vi "Regler Druck Kalter Block.vi"(7 "Index":i32, 8 "Fehler":errorcluster caption="Fehler (Eingang)") -> (0 "Fehler (Ausgang)":errorcluster)   [LabVIEW 2020, in "Regler.lvlib" / "Druckregler.lvlib"]
uses:
  Druckregler.lvlib
  Aktionen Param. Druckregler.ctl
  Aktionen Interne Werte.ctl
  Verwaltung/FGV IN Aktionen.ctl
  Konfig-Dateien/FGV Betriebsdaten Aktionen.ctl
  Verwaltung/FGV OUT Aktionen.ctl
  Allgemein/Aktionen FGV Dichtheitstest.ctl
  Allgemein/FGV Zustaende Aktionen.ctl
  Funktionstasten/Zustaende.ctl
  Allgemein/FGV Analysator aktiv.ctl
  Seiten/CalGas Aufschaltung/Auswahl Analysator.ctl
  Seiten/CalGas Aufschaltung/Auswahl Aufschaltpunkt.ctl
  Verwaltung/Verwaltung - cRIO.lvlib
  Visualisierungs Elemente/Zahlen-Eingabefeld.ctl
  Allgemein/Allgemein.lvlib
  Konfig-Dateien/Konfig-Dateien.lvlib
  Funktionstasten/Funktionstasten.lvlib
  Seiten/CalGas Aufschaltung/CalGas Aufschaltung.lvlib
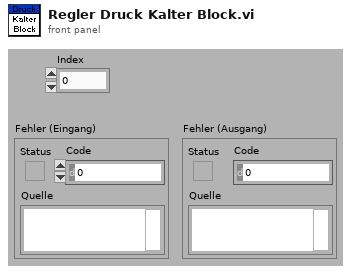
[diagram p1: front panel]
types:
  T1 = typedef "Regler.lvlib/Druckregler.lvlib/Aktionen Param. Druckregler.ctl" = enum16{"lesen", "schreiben", "Regler FT-IR", "Regler Ausgang", "Regler Durchfluss", "Regler PMA", "Regler NDIR", "Regler Filterblock", "Regler Gaskühler", "Regler Kalter Block"}
  T2 = typedef "Allgemein.lvlib/FGV Analysator aktiv.ctl" = enum16{"lesen", "Analysator", "CG Aufschaltung", "KAL Zustand", "AutaKal GT?"}
  T3 = typedef "Funktionstasten.lvlib/Zustaende.ctl" = enum16{"Standby", "Pause", "Eco", "Messen", "Kalibrieren", "Spülen Filter", "Spülen Leitung", "Umgebungsluft", "0-Gas", "Cal-Gas", "CG zu PNS", "-------------", "Init 1", "Init 2", "Init 3", "Init 4", "Messen vorbereiten", "Messen durchführen", "Exit"}
  T4 = typedef "Allgemein.lvlib/FGV Zustaende Aktionen.ctl" = enum16{"lesen", "Zustand PC", "Zustand cRIO", "Bildnummer", "Samplepoint", "Sysloglevel"}
  T5 = typedef "Allgemein.lvlib/Aktionen FGV Dichtheitstest.ctl" = enum16{"lesen", "schreiben"}
  T6 = typedef "Verwaltung - cRIO.lvlib/FGV OUT Aktionen.ctl" = enum16{"lesen", "ANA OUT", "DO 0-31", "DO 32-47"}
  T7 = typedef "Konfig-Dateien.lvlib/FGV Betriebsdaten Aktionen.ctl" = enum16{"lesen", "Anlagengrenzw.", "PID Param.", "Sonstige", "Sensor Para."}
  T8 = typedef "Verwaltung - cRIO.lvlib/FGV IN Aktionen.ctl" = enum16{"lesen", "DI", "AI", "Fühler Br.", "TC", "Fühler Br. TC"}
  T9 = typedef "Regler.lvlib/Druckregler.lvlib/Aktionen Interne Werte.ctl" = enum16{"lesen", "FT-IR", "Ausgang", "Pumpe", "laden", "speichern", "Änderung?", "Druck Kalter Block", "Dichtheitstest"}
  T10 = typedef "Status Analysatoren.lvlib/Status Analysatoren_Anzeige.ctl" = cluster{"FT-IR":bool, "FID":bool, "PMA":bool}
  T11 = typedef "Anlagengrenzwerte.lvlib/Anlagen-Grenzwerte Anzeige.ctl" = cluster{"Eingangsdruck FT-IR:":T12, "Durchfluss FT-IR:":T12, "Durchfluss CalGas:":T12, "Druck Ausgang:":T12, "Druck Kalter Block:":T12, "Heizleitungen intern:":T12, "Heizleitung zu FT-IR:":T12, "Heizung Filterblock:":T12, "Heizung Pumpe:":T12, "Heizleitung Extern SP1:":T12, "Heizleitung Extern SP2:":T12, "FT-IR Heizung Messzelle:":T12, "Schaltschranktemperatur:":T12, "Gaskühler:":T12}
  T12 = typedef "Anlagengrenzwerte.lvlib/Anlagen-Parameter Anzeige.ctl" = cluster{"Sollwert":sgl, "Warn-Min":sgl, "Warn-Max":sgl, "Abschalt-Min":sgl, "Abschalt-Max":sgl, "Regler":u16}
  T13 = typedef "Verwaltung - cRIO.lvlib/Analog Eingaenge.ctl" = cluster{"AI0: Durchfluss FT-IR":sgl, "AI1: Druck Ausgang":sgl, "AI2: Umgebungsdruck":sgl, "AI3: Druck FT-IR":sgl, "AI4: Druck CalGas":sgl, "AI5: Reserve":sgl, "AI6: Reserve":sgl, "AI7: Reserve":sgl, "Rohwert Durchfluss FT-IR":sgl, "Rohwert Druck Ausgang":sgl, "Rohwert Umgebungsdruck":sgl, "Rohwert Druck FT-IR":sgl, "Rohwert Druck CalGas":sgl, "Rohwert AI5":sgl, "Rohwert AI6":sgl, "Rohwert AI7":sgl, "Rohwert Diffdruck mbar FTIR":sgl}
  T14 = typedef "Verwaltung - cRIO.lvlib/Digital Ausgaenge 0-31.ctl" = cluster{"O0: Druckluft Versorgung":bool, "O1: CG 1 (FB Eingang 1)":bool, "O2: CG 2 (Kühlung FT-IR EIN)":bool, "O3: CG 3 (FB Bypass)":bool, "O4: CG 4 (FB CalGas)":bool, "O5: CG 5 (FB spülen/UL)":bool, "O6: CG 6 (FB zum FT-IR)":bool, "O7: CG 7 (FB zum FID)":bool, "O8: CG 8 (FB Reserve)":bool, "O9: (FB Reserve)":bool, "O10: (FB Umgebungsluft FID)":bool, "O11: (FB zum Gaskühler)":bool, "O12: FB Stickstoff zu FT-IR":bool, "O13: Optikbox FT-IR spülen":bool, "O14: (Purifier deaktivieren)":bool, "O15: (Umschaltung Purifier/Stickstoff)":bool, "O16: N2 Einblasung":bool, "O17: LSP LN2 Nachfüllung":bool, "O18: (Reserve)":bool, "O19: (Pumpe Eingang1)":bool, "O20: (Pumpe Eingang2)":bool, "O21: (Pumpe Spülen1)":bool, "O22: (Pumpe Spülen2)":bool, "O23: (Reserve)":bool, "O24: CalGas 1":bool, "O25: CalGas 2":bool, "O26: CG 3-8 (CalGas 3)":bool, "O27: Stickstoff aufschalten":bool, "O28: CG zu PNS":bool, "O29: FTIR Standby Spülung":bool, "O30: CG zu Entnahme(T90)":bool, "O31: (Purifier regenerieren)":bool}
  T15 = typedef "CalGas Aufschaltung.lvlib/Auswahl Aufschaltpunkt.ctl" = enum16{"über Filterblock", "Analysator direkt", "über PNS", "Entnahme", "Gasdivider"}
  T16 = typedef "CalGas Aufschaltung.lvlib/Auswahl Analysator.ctl" = enum16{"FT-IR", "FID", "PMA", "PMA/FID/FT-IR"}
  T17 = typedef "CalGas Aufschaltung.lvlib/Aufschaltung CalGas.ctl" = cluster{"Kalibriergas":T18, "Aufschaltpunkt":T15, "Analysator":T16}
  T18 = typedef "Auswahlfeld.ctl" = u16
  T19 = typedef "Zahlen-Eingabefeld.ctl" = sgl
  T20 = typedef "Verwaltung - cRIO.lvlib/Analog Eingaenge.ctl" = cluster{"AI0: Durchfluss FT-IR":sgl, "AI1: Druck Ausgang":sgl, "AI2: Umgebungsdruck":sgl, "AI3: Druck FT-IR":sgl, "AI4: Druck CalGas":sgl, "AI5: Taupunktsensor":sgl, "AI6: Reserve":sgl, "AI7: Druck CG PMA":sgl, "AI8: Durchfluss PMA":sgl, "AI9: Druck Kalter Block":sgl, "AI10: Umgebungsdruck(reserve)":sgl, "AI11: Temperatur Gaskühler":sgl, "AI12: Reserve":sgl, "AI13: Reserve":sgl, "AI14: Reserve":sgl, "AI15: Reserve":sgl, "Rohwert Durchfluss FT-IR":sgl, "Rohwert Druck Ausgang":sgl, "Rohwert Umgebungsdruck":sgl, "Rohwert Druck FT-IR":sgl, "Rohwert AI4":sgl, "Rohwert AI5":sgl, "Rohwert AI6":sgl, "Rohwert AI7":sgl, "Rohwert AI8":sgl, "Rohwert AI9":sgl, "Rohwert AI10":sgl, "Rohwert AI11":sgl, "Rohwert AI12":sgl, "Rohwert AI13":sgl, "Rohwert AI14":sgl, "Rohwert AI15":sgl, "Rohwert Diffdruck mbar FTIR":sgl}
  T21 = cluster{"Numerisch":sgl, "Numerisch":sgl, "Numerisch":sgl, "Numerisch":sgl, "Numerisch":sgl}
  T22 = typedef "Regler.lvlib/Druckregler.lvlib/Regler Interne Werte.ctl" = cluster{"PV":sgl, "D-action":sgl, "Error":sgl, "I-action":sgl, "OUT":sgl}
  T23 = typedef "Erweiterte Konfig.lvlib/Aktionen Dichtheitstest.ctl" = enum16{"Initialisieren", "Unterdruck aufbauen", "Prop schließen", "Warten", "Auswertung", "Fertig"}
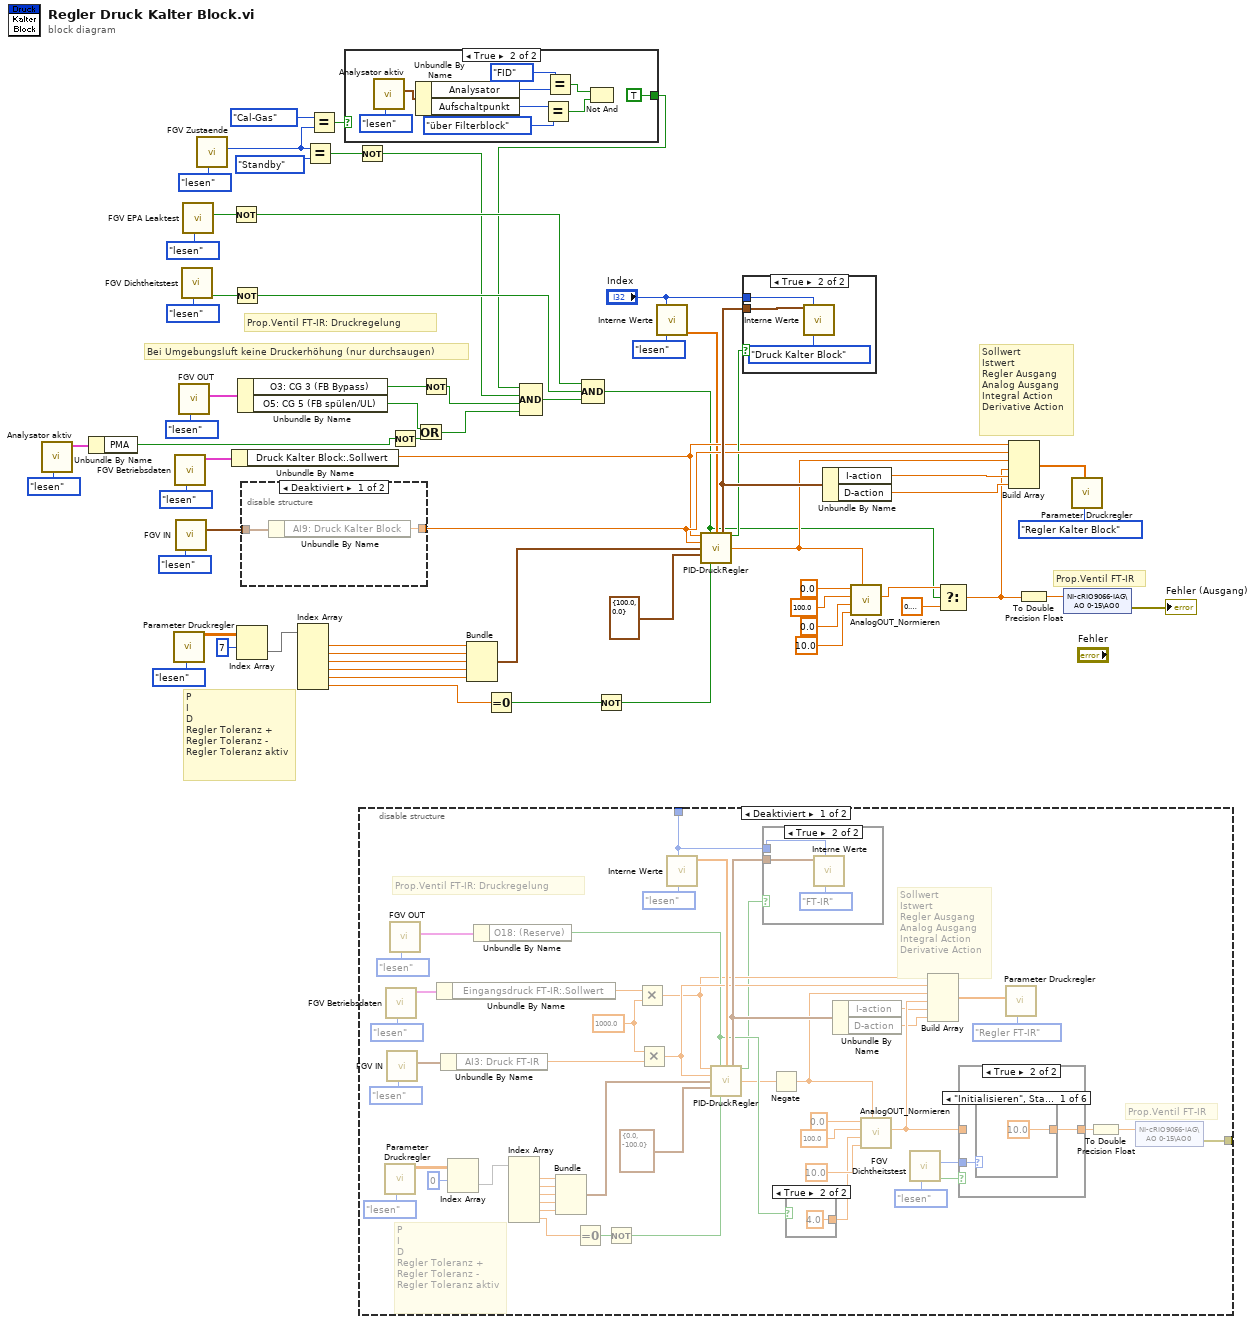
[diagram p0: block diagram]
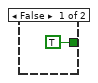
[diagram p3: hidden frame]
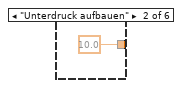
[diagram p7: hidden frame]
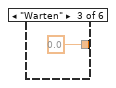
[diagram p8: hidden frame]
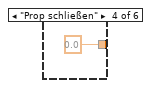
[diagram p9: hidden frame]
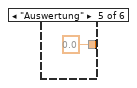
[diagram p10: hidden frame]
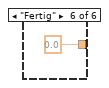
[diagram p11: hidden frame]
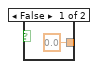
[diagram p12: hidden frame]
diagram:
  # "Bei Umgebungsluft keine Druckerhöhung (nur durchsaugen)"
  # "Prop.Ventil FT-IR"
  # "Prop.Ventil FT-IR: Druckregelung"
  # "Sollwert\nIstwert\nRegler Ausgang\nAnalog Ausgang\nIntegral Action\nDerivative Action"
  # "P\nI\nD\nRegler Toleranz +\nRegler Toleranz -\nRegler Toleranz aktiv"
  n1 = call "Analysator aktiv.vi"("Aktion"=FGV_Analysator_aktiv."lesen") -> ("Status Analysatoren"=w7:T10)  [unwired: 7 in, 3 out]
  n2 = Unbundle By Name(w7) -> ("PMA"=w3:bool)
  n3 = call "Parameter Druckregler.vi"("Aktionen"=Aktionen_Param._Druckregler."lesen") -> ("Regleparameter"=w48:sgl[][])  [unwired: 10 in, 8 out]
  n4 = call "FGV Betriebsdaten.vi"("Aktionen"=FGV_Betriebsdaten_Aktionen."lesen") -> ("Anlagen-Grenzwerte"=w34:T11)  [unwired: 7 in, 3 out]
  n5 = call "FGV IN.vi"("Aktion"=FGV_IN_Aktionen."lesen") -> ("Analog Eingänge"=w33:T13)  [unwired: 10 in, 4 out]
  n6 = call "FGV OUT.vi"("Aktion"=FGV_OUT_Aktionen."lesen") -> ("DO 0-31"=w35:T14)  [unwired: 7 in, 3 out]
  n7 = call "FGV Dichtheitstest.vi"("Aktionen"=Aktionen_FGV_Dichtheitstest."lesen") -> ("Dichtheitstest?"=w30:bool)  [unwired: 9 in, 1 out]
  n8 = call "FGV EPA Leaktest.vi"("Aktion"=enum16{"lesen", "schreiben"}."lesen") -> ("Leaktest aktiv"=w24:bool)  [unwired: 9 in, 1 out]
  n9 = call "FGV Zustaende.vi"("Aktionen"=FGV_Zustaende_Aktionen."lesen") -> ("Zustand cRIO"=w17:T3)  [unwired: 6 in, 4 out]
  n10 = Not(x=w24) -> (.not. x?=w23:bool)
  n11 = Not(x=w30) -> (.not. x?=w29:bool)
  n12 = Unbundle By Name(w34) -> ("Druck Kalter Block:.Sollwert"=w22:sgl)
  n13 = Index Array(array=w48, index (row)=7 ("Deaktivierter Index (Spalte)")) -> (element=w47:sgl[])  [unwired: 1 in]
  n14 = Unbundle By Name(w35) -> ("O3: CG 3 (FB Bypass)"=w27:bool, "O5: CG 5 (FB spülen/UL)"=w5:bool)
  n15 = disable-structure shown="Deaktiviert" {
    disable-tunnel: [w67 _] -> w45
    disable-tunnel: w33 -> [w66 _]
    frame Disabled {
      n16 = Unbundle By Name(w66) -> ("AI9: Druck Kalter Block"=w67:sgl)
    }
    frame Enabled {
    }
  }
  n17 = Index Array(array=w47) -> (element #1=w58:sgl, element #2=w57:sgl, element #3=w56:sgl, element #4=w55:sgl, element #5=w54:sgl, element #6=w43:sgl)  [unwired: 6 in]
  n18 = Equal?(x=w17, y=Zustaende."Standby") -> (x = y?=w18:bool)
  n19 = Equal?(x=Zustaende."Cal-Gas", y=w17) -> (x = y?=w15:bool)
  n20 = case shown="True" w15 {
    tunnel: [TRUE TRUE] -> w14
    frame False {
    }
    frame True {
      n21 = call "Analysator aktiv.vi"("Aktion"=FGV_Analysator_aktiv."lesen") -> ("Aufschaltung CalGas"=w77:T17)  [unwired: 7 in, 3 out]
      n22 = Unbundle By Name(w77) -> ("Analysator"=w74:T16, "Aufschaltpunkt"=w75:T15)
      n23 = Equal?(x=w75, y=Auswahl_Aufschaltpunkt."über Filterblock") -> (x = y?=w70:bool)
      n24 = Equal?(x=Auswahl_Analysator."FID", y=w74) -> (x = y?=w71:bool)
      n25 = Not And(1:w70, 2:w71) -> ()  [unwired: 1 out]
    }
  }
  n26 = Not(x=w18) -> (.not. x?=w19:bool)
  n27 = disable-structure shown="Deaktiviert" {
    disable-tunnel: _ -> [w88 _]
    disable-tunnel: [w84 _] -> _
    frame Disabled {
      w103 = T19 1000.0 ("y")
      # "Prop.Ventil FT-IR"
      # "Prop.Ventil FT-IR: Druckregelung"
      # "Sollwert\nIstwert\nRegler Ausgang\nAnalog Ausgang\nIntegral Action\nDerivative Action"
      # "P\nI\nD\nRegler Toleranz +\nRegler Toleranz -\nRegler Toleranz aktiv"
      n28 = call "Parameter Druckregler.vi"("Aktionen"=Aktionen_Param._Druckregler."lesen") -> ("Regleparameter"=w108:sgl[][])  [unwired: 7 in, 3 out]
      n29 = call "FGV Betriebsdaten.vi"("Aktionen"=FGV_Betriebsdaten_Aktionen."lesen") -> ("Anlagen-Grenzwerte"=w79:T11)  [unwired: 7 in, 3 out]
      n30 = call "FGV IN.vi"("Aktion"=FGV_IN_Aktionen."lesen") -> ("Analog Eingänge"=w78:T20)  [unwired: 8 in, 2 out]
      n31 = call "FGV OUT.vi"("Aktion"=FGV_OUT_Aktionen."lesen") -> ("DO 0-31"=w80:T14)  [unwired: 7 in, 3 out]
      n32 = Unbundle By Name(w79) -> ("Eingangsdruck FT-IR:.Sollwert"=w104:sgl)
      n33 = Unbundle By Name(w78) -> ("AI3: Druck FT-IR"=w102:sgl)
      n34 = Index Array(array=w108, index (row)=0 ("Deaktivierter Index (Spalte)")) -> (element=w107:sgl[])  [unwired: 1 in]
      n35 = Unbundle By Name(w80) -> ("O18: (Reserve)"=w93:bool)
      n36 = Index Array(array=w107) -> (element #1=w119:sgl, element #2=w118:sgl, element #3=w117:sgl, element #4=w116:sgl, element #5=w115:sgl, element #6=w90:sgl)  [unwired: 6 in]
      n37 = Bundle("Numerisch"=w119, "Numerisch"=w118, "Numerisch"=w117, "Numerisch"=w116, "Numerisch"=w115) -> (w113:T21)  [unwired: 1 in]
      n38 = Equal To 0?(x=w90) -> (x = 0?=w114:bool)
      n39 = Not(x=w114) -> (.not. x?=w112:bool)
      n40 = Multiply(x=w104, y=w103) -> (x*y=w92:T19)
      n41 = Multiply(x=w103, y=w102) -> (x*y=w101:T19)
      n42 = call "Interne Werte.vi"("Aktionen Interne Werte"=Aktionen_Interne_Werte."lesen", "Index"=w88) -> ("FT-IR"=w125:sgl[])  [unwired: 4 in, 5 out]
      n43 = call "PID-DruckRegler.vi"("Sollwert"=w92, "Regler EIN"=w93, "Regler Interne Werte"=w125, "Istwert"=w101, "PID-Parameter"=w113, "output range"=cluster{"output high":dbl, "output low":dbl} {"output high"=0.0, "output low"=-100.0}, "Regler Toleranz verwenden?"=w112) -> ("Regler Interne Werte"=w124:T22, "Interne Werte speichern"=w87:bool, "Output"=w91:sgl)  [unwired: 6 in]
      n44 = case shown="True" w87 {
        tunnel: w88 -> [_ w127]
        tunnel: w124 -> [_ w126]
        frame False {
        }
        frame True {
          n45 = call "Interne Werte.vi"("Aktionen Interne Werte"=Aktionen_Interne_Werte."FT-IR", "Index"=w127, "Regler Interne Werte"=w126) -> ()  [unwired: 3 in, 6 out]
        }
      }
      n46 = Negate(x=w91) -> (-x=w94:sgl)
      n47 = case shown="True" w93 {
        tunnel: [sgl 0.0 ("Untergrenze") sgl 4.0 ("Untergrenze")] -> w111
        frame False {
        }
        frame True {
        }
      }
      n48 = Unbundle By Name(w124) -> ("I-action"=w86:sgl, "D-action"=w85:sgl)
      n49 = call "AnalogOUT_Normieren.vi"("Analogwert"=w94, "Obergrenze"=sgl 10.0, "Untergrenze"=w111, "Max Analogwert"=sgl 100.0, "Min Analogwert"=sgl 0.0) -> ("Normierter Wert"=w98:sgl)  [unwired: 6 in]
      n50 = call "FGV Dichtheitstest.vi"("Aktionen"=Aktionen_FGV_Dichtheitstest."lesen") -> ("Dichtheitstest?"=w95:bool, "Aktionen Dichtheitstest"=w96:T23)  [unwired: 9 in]
      n51 = Build Array(w92, w101, w94, w98, w86, w85) -> (w106:T19[])
      n52 = case shown="True" w95 {
        tunnel: w96 -> [_ w131]
        tunnel: w98 -> [w129 _]
        tunnel: [w129 w130] -> w97
        frame False {
        }
        frame True {
          n53 = case shown="\"Initialisieren\", Standard" w131 {
            tunnel: [sgl 10.0 ("Untergrenze") sgl 10.0 ("Untergrenze") sgl 0.0 ("Untergrenze") sgl 0.0 ("Untergrenze") sgl 0.0 ("Untergrenze") sgl 0.0 ("Untergrenze")] -> w130
            frame "Initialisieren", Default {
            }
            frame "Unterdruck aufbauen" {
            }
            frame "Warten" {
            }
            frame "Prop schließen" {
            }
            frame "Auswertung" {
            }
            frame "Fertig" {
            }
          }
        }
      }
      n54 = call "Parameter Druckregler.vi"("Aktionen"=Aktionen_Param._Druckregler."Regler FT-IR", "Werte FT-IR"=w106) -> ()  [unwired: 6 in, 4 out]
      n55 = To Double Precision Float(number=w97) -> (double precision float=w100:dbl)
      n56 = shared-variable "NI-cRIO9066-IAG\\AO 0-15\\AO0"(w100) -> (error out=w84:errorcluster)  [unwired: 1 in]
    }
    frame Enabled {
    }
  }
  n57 = Not(x=w3) -> (.not. x?=w6:bool)
  n58 = Or(x=w5, y=w6) -> (x .or. y?=w4:bool)
  n59 = Not(x=w27) -> (.not. x?=w26:bool)
  n60 = Bundle("Numerisch"=w58, "Numerisch"=w57, "Numerisch"=w56, "Numerisch"=w55, "Numerisch"=w54) -> (w52:T21)  [unwired: 1 in]
  n61 = Equal To 0?(x=w43) -> (x = 0?=w53:bool)
  n62 = Compound Arithmetic op=AND ("Mehrfacharithmetik")(w14, w19, w26, w4) -> (w28:bool)
  n63 = Compound Arithmetic op=AND ("Mehrfacharithmetik")(w23, w29, w28) -> (w10:bool)
  n64 = Not(x=w53) -> (.not. x?=w51:bool)
  n65 = call "Interne Werte.vi"("Index"="Index", "Aktionen Interne Werte"=Aktionen_Interne_Werte."lesen") -> ("Druck Kalter Block"=w13:sgl[])  [unwired: 7 in, 6 out]
  n66 = call "PID-DruckRegler.vi"("Sollwert"=w22, "Regler EIN"=w10, "Regler Interne Werte"=w13, "Istwert"=w45, "PID-Parameter"=w52, "output range"=cluster{"output high":dbl, "output low":dbl} {"output high"=100.0, "output low"=0.0}, "Regler Toleranz verwenden?"=w51) -> ("Regler Interne Werte"=w63:T22, "Interne Werte speichern"=w41:bool, "Output"=w32:sgl)  [unwired: 6 in]
  n67 = case shown="True" w41 {
    tunnel: "Index" -> [_ w141]
    tunnel: w63 -> [_ w140]
    frame False {
    }
    frame True {
      n68 = call "Interne Werte.vi"("Regler Interne Werte"=w140, "Index"=w141, "Aktionen Interne Werte"=Aktionen_Interne_Werte."Druck Kalter Block") -> ()  [unwired: 6 in, 7 out]
    }
  }
  n69 = Unbundle By Name(w63) -> ("I-action"=w40:sgl, "D-action"=w39:sgl)
  n70 = call "AnalogOUT_Normieren.vi"("Analogwert"=w32, "Obergrenze"=sgl 10.0, "Untergrenze"=sgl 0.0, "Max Analogwert"=sgl 100.0, "Min Analogwert"=sgl 0.0) -> ("Normierter Wert"=w12:sgl)  [unwired: 6 in]
  n71 = Select(t=w12, s=w10, f=sgl 0.2) -> (s? t:f=w9:sgl)
  n72 = Build Array(w22, w45, w32, w9, w40, w39) -> (w1:sgl[])
  n73 = To Double Precision Float(number=w9) -> (double precision float=w44:dbl)
  n74 = shared-variable "NI-cRIO9066-IAG\\AO 0-15\\AO0"(w44) -> (error out=→"Fehler (Ausgang)":errorcluster)  [unwired: 1 in]
  n75 = call "Parameter Druckregler.vi"("Werte Kalter Block"=w1, "Aktionen"=Aktionen_Param._Druckregler."Regler Kalter Block") -> ()  [unwired: 9 in, 9 out]
